vi "Initialize5WirexVDTParameters.vi"(6 "Specified Channel Ref List":T1[](array[typedef]) format="%.0x", 8 "error in":errorcluster, 9 "FPGA Session In":refnum<class "FPGA Interface Base.lvclass">, 11 "Device Reference in":T1 format="%.0x") -> (0 "error out":errorcluster, 1 "FPGA Session Out":refnum<class "FPGA Interface Base.lvclass">, 2 "5 Wire xVDT Parameters":T2[](array[typedef]), 3 "Device Reference out":T1 format="%.0x")   [LabVIEW 2011, in "Sensor Simulation Custom Device.lvlib"]
uses:
  Sensor Simulation Custom Device.lvlib
  <vilib>/NI Veristand/Custom Device API/Custom Device Item Ref.ctl
  TypeDefs/5 Wire xVDT Parameters.ctl
  <userlib>/_FPGA Interface Advanced Tools/FPGA Interface Base/FPGA Interface Base.lvclass
  TypeDefs/SensorType.ctl
  System Explorer/TypeDefs/xVDT.ctl
  <vilib>/rvi/DataTransferAndStorage/Container/Common/niFpgaDataTypeControl.ctl
  <userlib>/_FPGA Interface Advanced Tools/FPGA Interface Base/FPGA Interface Base.lvclass/FPGA Interface Base.ctl
  <vilib>/NI Veristand/Custom Device Tools/Custom Device Utility Library/NI VeriStand - Search for All Items by Property.vi
  Global.vi
  <vilib>/NI Veristand/Custom Device API/Get Item Property (Variant).vi
  <vilib>/NI Veristand/Custom Device API/Get Item Property (Double).vi
  <vilib>/Utility/error.llb/Error Cluster From Error Code.vi
  <vilib>/NI Veristand/Custom Device API/Custom Device API.lvlib
  <vilib>/NI Veristand/Custom Device Tools/Custom Device Utility Library/Custom Device Utility Library.lvlib
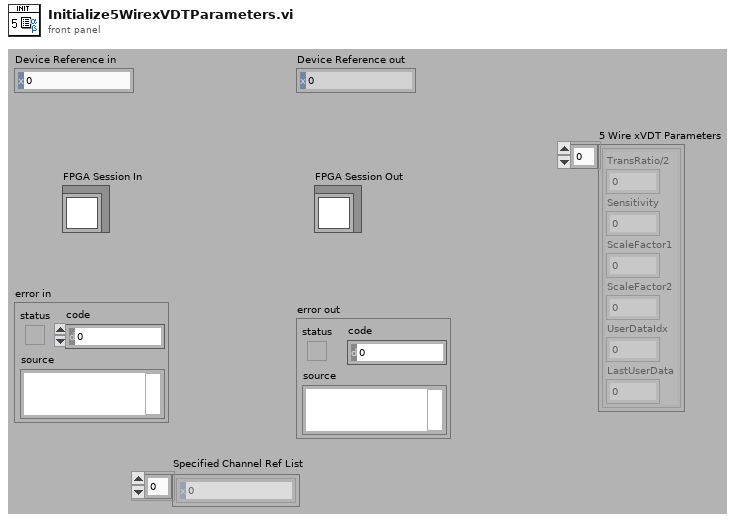
[diagram p1: front panel]
types:
  T1 = typedef "Custom Device API.lvlib/Custom Device Item Ref.ctl" = u64
  T2 = typedef "Sensor Simulation Custom Device.lvlib/5 Wire xVDT Parameters.ctl" = cluster{"TransRatio/2":dbl, "Sensitivity":dbl, "ScaleFactor1":u32, "ScaleFactor2":u32, "UserDataIdx":i32, "LastUserData":dbl}
  T3 = typedef "Sensor Simulation Custom Device.lvlib/SensorType.ctl" = enum16{"Resolver", "4 Wire xVDT", "5 Wire xVDT", "Invalid"}
  T4 = typedef "niFpgaDataTypeControl.ctl" = enum32{"Boolean", "I8", "I16", "I32", "I64", "U8", "U16", "U32", "U64", "FXP", "CustomControl"}
  T5 = typedef "Sensor Simulation Custom Device.lvlib/xVDT.ctl" = cluster{"ScaleFactor 1":string, "ScaleFactor 2":string, "#":string}
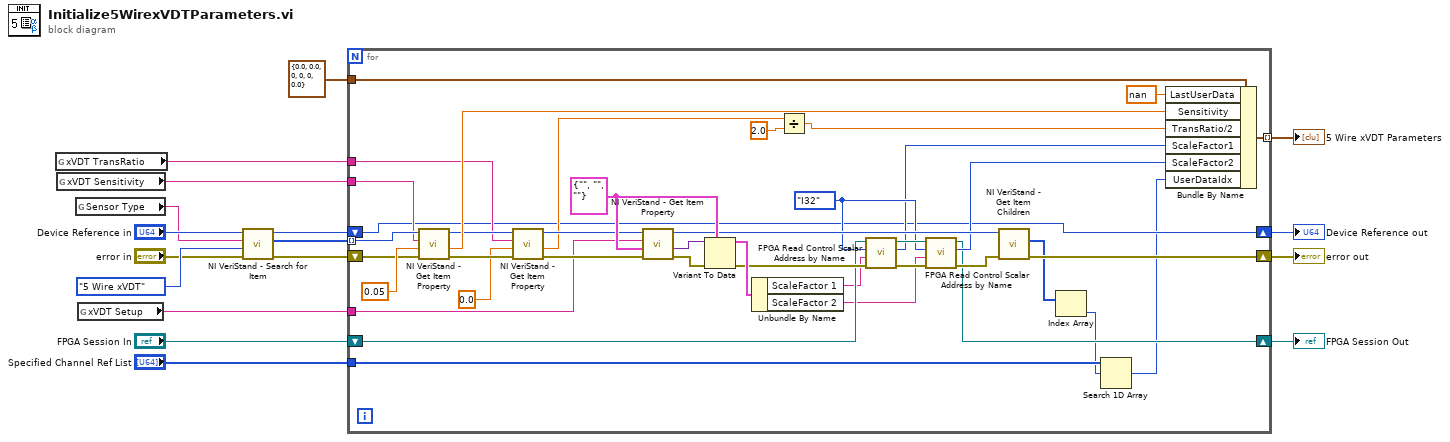
[diagram p0: block diagram]
diagram:
  n1 = global read "Global.vi" "xVDT TransRatio"() -> (w5:string)
  n2 = global read "Global.vi" "xVDT Sensitivity"() -> (w6:string)
  n3 = global read "Global.vi" "Sensor Type"() -> (w15:string)
  n4 = global read "Global.vi" "xVDT Setup"() -> (w4:string)
  n5 = call-poly <vilib>:"NI VeriStand - Search for Item.vi"("error in"="error in", "Property Value"=SensorType."5 Wire xVDT" ("Sensor"), "Property Name"=w15, "Section Ref in"="Device Reference in") -> ("error out"=w10:errorcluster, "Item Refs"=w9:T1[], "Section Ref out"=w8:T1)  [unwired: 4 in, 1 out]
  n6 = for {
    shift-right: [w26] -> w17
    shift-left: w10 -> [w56]
    tunnel: w9 -> [w55] mode=indexing
    tunnel: T2 {"TransRatio/2"=0.0, "Sensitivity"=0.0, "ScaleFactor1"=0, "ScaleFactor2"=0, "UserDataIdx"=0, "LastUserData"=0.0} ("4 Wire LVDT Parameters") -> [w49]
    tunnel: [w47] -> w13 mode=indexing
    shift-right: [w25] -> w12
    shift-left: w8 -> [w25]
    tunnel: w6 -> [w40]
    tunnel: w5 -> [w39]
    tunnel: w4 -> [w38]
    shift-right: [w27] -> w2
    shift-left: "FPGA Session In" -> [w33]
    tunnel: "Specified Channel Ref List" -> [w23]
    w30 = niFpgaDataTypeControl."I32" ("Data Type")
    w52 = T5 {"ScaleFactor 1"="", "ScaleFactor 2"="", "#"=""} ("xVDT")
    n7 = call-poly <vilib>:"NI VeriStand - Get Item Property.vi"("error in (no error)"=w56, "Default Value"=0.05, "Property Name"=w40, "Item Ref in"=w55) -> ("error out"=w44:errorcluster, "Value"=w48:dbl, "Item Ref out"=w46:T1)  [unwired: 4 in, 1 out]
    n8 = call-poly <vilib>:"NI VeriStand - Get Item Property.vi"("error in (no error)"=w44, "Default Value"=0.0, "Property Name"=w39, "Item Ref in"=w46) -> ("error out"=w43:errorcluster, "Value"=w41:dbl, "Item Ref out"=w45:T1)  [unwired: 4 in, 1 out]
    n9 = call-poly <vilib>:"NI VeriStand - Get Item Property.vi"("error in (no error)"=w43, "Default Value"=w52, "Property Name"=w38, "Item Ref in"=w45) -> ("error out"=w54:errorcluster, "Value"=w53:variant, "Item Ref out"=w50:T1)  [unwired: 4 in, 1 out]
    n10 = Variant To Data(error in=w54, type=w52, Variant=w53) -> (data=w51:T5, error out=w37:errorcluster)
    n11 = Unbundle By Name(w51) -> ("ScaleFactor 1"=w32:string, "ScaleFactor 2"=w31:string)
    n12 = Divide(x=w41, y=2.0 ("x")) -> (x/y=w19:dbl)
    n13 = call <userlib>:"FPGA Read Control Scalar Address by Name.vi"("error in (no error)"=w37, "Name"=w32, "Data Type"=w30, "FPGA Interface Base in"=w33) -> ("error out"=w36:errorcluster, "Address"=w29:u32, "FPGA Interface Base out"=w35:refnum<class "FPGA Interface Base.lvclass">)  [unwired: 4 in, 1 out]
    n14 = call <userlib>:"FPGA Read Control Scalar Address by Name.vi"("error in (no error)"=w36, "Name"=w31, "Data Type"=w30, "FPGA Interface Base in"=w35) -> ("error out"=w34:errorcluster, "Address"=w28:u32, "FPGA Interface Base out"=w27:refnum<class "FPGA Interface Base.lvclass">)  [unwired: 4 in, 1 out]
    n15 = call <vilib>:"NI VeriStand - Get Item Children.vi"("error in (no error)"=w34, "Item Ref in"=w50) -> ("error out"=w26:errorcluster, "Child Refs"=w24:T1[])  [unwired: 6 in, 2 out]
    n16 = Index Array(array=w24) -> (element=w22:T1)  [unwired: 1 in]
    n17 = Search 1D Array(1D array=w23, element=w22) -> (index of element=w21:i32)  [unwired: 1 in]
    n18 = Bundle By Name(cluster=w49, "LastUserData"=nan, "Sensitivity"=w48, "TransRatio/2"=w19, "ScaleFactor1"=w29, "ScaleFactor2"=w28, "UserDataIdx"=w21) -> (w47:T2)
  }
  "error out" <- w17
  "Device Reference out" <- w12
  "5 Wire xVDT Parameters" <- w13
  "FPGA Session Out" <- w2
